vi "navX Example v2.vi"() -> ()   [LabVIEW 2015]
uses:
  navX Library v2/TypeDefs/Flags/Z900_navX_Flags_HardwareRevTypeDef.ctl
  navX Library v2/TypeDefs/Flags/Z900_navX_Flags_OmnimountConfigTypeDef.ctl
  navX Library v2/TypeDefs/Z900_navX_SerialStreamTypeDef.ctl
  NI WPI/WPI_SerialPort_USB.ctl
  <vilib>/Rock Robotics/SystemInterfaces/i2clib/i2c_bus.ctl
  <vilib>/Rock Robotics/SystemInterfaces/spilib/spi_bus.ctl
  navX Library v2/TypeDefs/Flags/Z900_navX_Flags_OpStatusTypeDef.ctl
  navX Library v2/TypeDefs/Flags/Z900_navX_Flags_CalibrationStatusTypeDef.ctl
  navX Library v2/IO/Open/Z900_navX_Open_Serial.vi
  navX Library v2/IO/Open/Z900_navX_Open_I2C.vi
  navX Library v2/IO/Open/Z900_navX_Open_SPI.vi
  navX Library v2/navX Library v2.lvlib
  NI WPI/NI WPI Serial USB.lvlib
panel:
  in  "Zero Displacement":bool
  out "Status":T3 {"OP Status" items=["INITIALIZING", "SELFTEST_IN_PROGRESS", "ERROR", "IMU_AUTOCAL_IN_PROGRESS", "NORMAL"]; "Calibration Status" items=["IMU_CAL_STATE_MASK"=3, "IMU_CAL_STATE_INPROGRESS"=0, "IMU_CAL_STATE_ACCUMULATE"=1, "IMU_CAL_STATE_COMPLETE"=2]}
  out "Connected":bool
  out "ERROR!":bool
  in  "Enable Logs":bool
  in  "Clear Log":bool
  out "Internal Error Log":errorcluster[](array[cluster])
  out "Log Size":i32
  in  "Interface Control":enum32{"Serial", "I2C", "SPI"}(tab)
  in  "Serial Port":T4=enum."MXP TTL"
  in  "Update Stream Type":bool
  in  "Stream Type":T5=enum."AHRS"
  in  "I2C Bus":T6=enum."I2C MXP"
  in  "SPI Bus":T7=enum."SPI MXP"
  in  "Clock Rate (Hz)":dbl=2000000.0 format="%_6f"
  in  "Zero Yaw":bool
  out "Raw Values":T8
  out "Quaternion":T9
  out "Linear Acceleration":T10
  out "Displacement":T11
  out "Offsets":T12
  out "Timestamp":u32
  out "MPUTemp":dbl(slide) scale=20.0..50.0
  in  "Update Rate":u8=50 min=4 max=60
  out "Board Information":T15 {"Board"."Hardware Revision" items=["navX-MXP"=33, "navX-Micro"=40]; "Omnimount Config" items=["DEFAULT", "X_UP", "X_DOWN", "Y_UP", "Y_DOWN", "Z_UP", "Z_DOWN"]}
  out "YRPHfH":T16
  in  "stop":bool
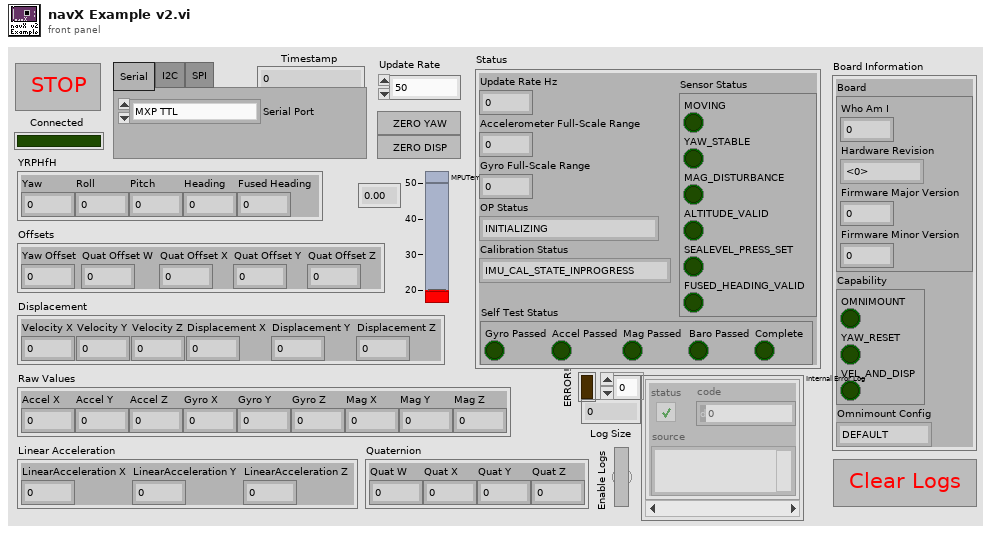
[diagram p1: front panel]
types:
  T1 = typedef "navX Library v2.lvlib/Z900_navX_Flags_OpStatusTypeDef.ctl" = u8
  T2 = typedef "navX Library v2.lvlib/Z900_navX_Flags_CalibrationStatusTypeDef.ctl" = u8
  T3 = cluster{"Update Rate Hz":u8, "Accelerometer Full-Scale Range":u8, "Gyro Full-Scale Range":u16, "OP Status":T1, "Calibration Status":T2, "Sensor Status":cluster{"MOVING":bool, "YAW_STABLE":bool, "MAG_DISTURBANCE":bool, "ALTITUDE_VALID":bool, "SEALEVEL_PRESS_SET":bool, "FUSED_HEADING_VALID":bool}, "Self Test Status":cluster{"Gyro Passed":bool, "Accel Passed":bool, "Mag Passed":bool, "Baro Passed":bool, "Complete":bool}}
  T4 = typedef "NI WPI Serial USB.lvlib/WPI_SerialPort_USB.ctl" = enum16{"Onboard RS-232", "MXP TTL", "USB"}
  T5 = typedef "navX Library v2.lvlib/Z900_navX_SerialStreamTypeDef.ctl" = enum16{"YRPH", "Quaterinons", "Gyro/Raw", "AHRS", "AHRSAndPositioning"}
  T6 = typedef "i2c_bus.ctl" = enum16{"I2C On-Board", "I2C MXP", "Invalid"}
  T7 = typedef "spi_bus.ctl" = enum16{"SPI On-Board, CS0", "SPI On-Board, CS1", "SPI On-Board, CS2", "SPI On-Board, CS3", "SPI MXP", "Invalid"}
  T8 = cluster{"Accel X":dbl, "Accel Y":dbl, "Accel Z":dbl, "Gyro X":dbl, "Gyro Y":dbl, "Gyro Z":dbl, "Mag X":dbl, "Mag Y":dbl, "Mag Z":dbl}
  T9 = cluster{"Quat W":dbl, "Quat X":dbl, "Quat Y":dbl, "Quat Z":dbl}
  T10 = cluster{"LinearAcceleration X":dbl, "LinearAcceleration Y":dbl, "LinearAcceleration Z":dbl}
  T11 = cluster{"Velocity X":dbl, "Velocity Y":dbl, "Velocity Z":dbl, "Displacement X":dbl, "Displacement Y":dbl, "Displacement Z":dbl}
  T12 = cluster{"Yaw Offset":dbl, "Quat Offset W":dbl, "Quat Offset X":dbl, "Quat Offset Y":dbl, "Quat Offset Z":dbl}
  T13 = typedef "navX Library v2.lvlib/Z900_navX_Flags_HardwareRevTypeDef.ctl" = u8
  T14 = typedef "navX Library v2.lvlib/Z900_navX_Flags_OmnimountConfigTypeDef.ctl" = u8
  T15 = cluster{"Board":cluster{"Who Am I":u8, "Hardware Revision":T13, "Firmware Major Version":u8, "Firmware Minor Version":u8}, "Capability":cluster{"OMNIMOUNT":bool, "YAW_RESET":bool, "VEL_AND_DISP":bool}, "Omnimount Config":T14}
  T16 = cluster{"Yaw":dbl, "Roll":dbl, "Pitch":dbl, "Heading":dbl, "Fused Heading":dbl}
  T17 = cluster{"Interface Control":enum32{"Serial", "I2C", "SPI"}, "Serial Port":T4, "I2C Bus":T6, "SPI Bus":T7, u8, "Clock Rate (Hz)":dbl}
  T18 = cluster{"Interface Control":bool, "Serial Port":bool, "I2C Bus":bool, "SPI Bus":bool, bool, "Clock Rate (Hz)":bool}
  T19 = typedef "navX Library v2.lvlib/Z900_navX_DeviceTypeDef.ctl" = cluster{"Interface":cluster{"Protocol":T20, "Update Rate (4Hz-100Hz)":u8, "navX Open TypeDef":variant}, "Notify Packet":refnum<notifier>, "Loop VI Refnum":refnum<vi>, "Ready to Close Occurrence Refnum":refnum<k4>}
  T20 = typedef "navX Library v2.lvlib/Z900_navX_ProtocolTypeDef.ctl" = enum16{"SERIAL", "I2C", "SPI"}
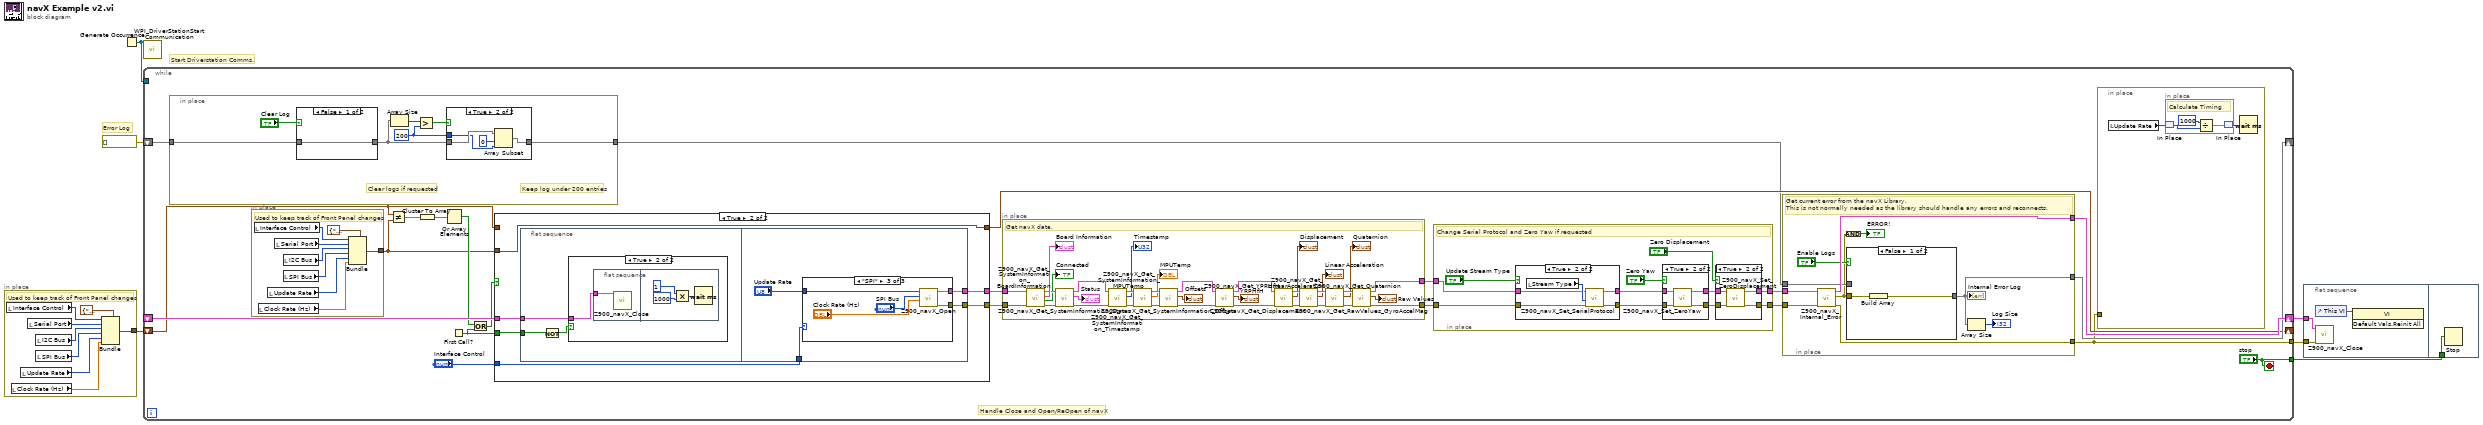
[diagram p0: block diagram]
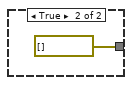
[diagram p3: hidden frame]
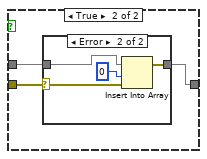
[diagram p4: hidden frame]
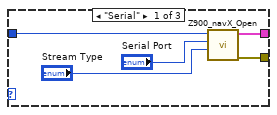
[diagram p11: hidden frame]
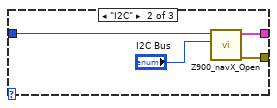
[diagram p12: hidden frame]
diagram:
  # "Start Driverstation Comms."
  # "Error Log"
  n1 = in-place {
    in-place-border: [w13] -> w3
    # "Used to keep track of Front Panel changes"
    n2 = local read "Interface Control"() -> (w12:enum32{"Serial", "I2C", "SPI"})
    n3 = local read "Clock Rate (Hz)"() -> (w7:dbl)
    n4 = local read "Update Rate"() -> (w8:u8)
    n5 = local read "Serial Port"() -> (w11:T4)
    n6 = local read "I2C Bus"() -> (w10:T6)
    n7 = local read "SPI Bus"() -> (w9:T7)
    n8 = Bundle(cluster=T17 {"Interface Control"=enum."Serial", "Serial Port"=enum."Onboard RS-232", "I2C Bus"=enum."I2C On-Board", "SPI Bus"=enum."SPI On-Board, CS0", 0, "Clock Rate (Hz)"=0.0} ("output cluster"), "Interface Control"=w12, "Serial Port"=w11, "I2C Bus"=w10, "SPI Bus"=w9, w8, "Clock Rate (Hz)"=w7) -> (w13:T17)
  }
  n9 = Generate Occurrence() -> (w2:refnum<k4>)
  n10 = call <vilib>:"WPI_DriverStationStart Communication.vi"("occurrence"=w2) -> ()  [unwired: 11 in]
  n11 = while {
    shift-right: [w32] -> w6
    shift-left: _ -> [w30]
    shift-right: [w31] -> _
    shift-left: errorcluster[] [] -> [w18]
    tunnel: [w15] -> w4
    shift-right: [w21] -> _
    shift-left: w3 -> [w20]
    tunnel: w2 -> [_]
    tunnel: ["stop"] -> w1
    stop <- "stop" stop-if-true
    # "Handle Close and Open/ReOpen of navX"
    n12 = in-place {
      in-place-border: w18 -> [w56]
      in-place-border: [w52] -> w17
      w51 = 200 ("y")
      # "Clear logs if requested"
      # "Keep log under 200 entries"
      n13 = case shown="False" "Clear Log" {
        tunnel: [w62 errorcluster[] []] -> w50
        tunnel: w56 -> [w62 _]
        frame False {
        }
        frame True {
        }
      }
      n14 = Array Size(array=w50) -> (size(s)=w55:i32)
      n15 = Greater?(x=w55, y=w51) -> (0:w53:bool)
      n16 = case shown="True" w53 {
        tunnel: [w57 w58] -> w52
        tunnel: w50 -> [w57 w61]
        tunnel: w51 -> [_ w59]
        frame False {
        }
        frame True {
          n17 = Array Subset(array=w61, index=0, length=w59) -> (w58:errorcluster[])
        }
      }
    }
    n18 = in-place {
      in-place-border: [w48] -> w16
      # "Used to keep track of Front Panel changes"
      n19 = local read "Interface Control"() -> (w47:enum32{"Serial", "I2C", "SPI"})
      n20 = local read "Clock Rate (Hz)"() -> (w42:dbl)
      n21 = local read "Update Rate"() -> (w43:u8)
      n22 = local read "Serial Port"() -> (w46:T4)
      n23 = local read "I2C Bus"() -> (w45:T6)
      n24 = local read "SPI Bus"() -> (w44:T7)
      n25 = Bundle(cluster=T17 {"Interface Control"=enum."Serial", "Serial Port"=enum."Onboard RS-232", "I2C Bus"=enum."I2C On-Board", "SPI Bus"=enum."SPI On-Board, CS0", 0, "Clock Rate (Hz)"=0.0} ("output cluster"), "Interface Control"=w47, "Serial Port"=w46, "I2C Bus"=w45, "SPI Bus"=w44, w43, "Clock Rate (Hz)"=w42) -> (w48:T17)
    }
    n26 = Not Equal?(x=w20, y=w16) -> (x != y?=w24:T18)
    n27 = Cluster To Array(cluster=w24) -> (array=w23:bool[])
    n28 = Or Array Elements(Boolean array=w23) -> (logical OR=w22:bool)
    n29 = First Call?() -> (First Call?: T/F=w26:bool)
    n30 = Or(x=w22, y=w26) -> (x .or. y?=w27:bool)
    n31 = case shown="True" w27 {
      tunnel: w30 -> [w148 w154]
      tunnel: [w148 w149] -> w29
      tunnel: [_ w153] -> w28
      tunnel: "Interface Control" -> [_ w152]
      tunnel: w26 -> [_ w151]
      tunnel: w16 -> [_ w150]
      tunnel: [w147 w150] -> w21
      tunnel: w20 -> [w147 _]
      frame False {
      }
      frame True {
        n32 = flat-sequence {
          tunnel: w151 -> [w155]
          tunnel: w154 -> [w156]
          tunnel: [w165] -> w149
          tunnel: [w164] -> w153
          tunnel: w152 -> [w163]
          frame #0 {
            n33 = Not(x=w155) -> (.not. x?=w157:bool)
            n34 = case shown="True" w157 {
              tunnel: w156 -> [_ w158]
              frame False {
              }
              frame True {
                n35 = flat-sequence {
                  tunnel: w158 -> [w159]
                  frame #0 {
                    n36 = call "Z900_navX_Close.vi"("navX Device"=w159) -> ()  [unwired: 10 in, 1 out]
                  }
                  frame #1 {
                    n37 = Multiply(x=u32 1, y=u32 1000 ("x")) -> (x*y=w161:u32)
                    n38 = Wait (ms)(milliseconds to wait=w161) -> ()  [unwired: 1 out]
                  }
                }
              }
            }
          }
          frame #1 {
            n39 = case shown="\"SPI\"" w163 {
              tunnel: [w169 w173 w179] -> w165
              tunnel: [w168 w172 w178] -> w164
              tunnel: "Update Rate" -> [w167 w175 w177]
              frame "Serial" {
                n40 = call-poly "Z900_navX_Open.vi"("Stream Type"="Stream Type", "Serial Port"="Serial Port", "Update Rate (4Hz-60Hz)"=w167) -> ("error out"=w168:errorcluster, "navX Device"=w169:T19)  [unwired: 7 in]
              }
              frame "I2C" {
                n41 = call-poly "Z900_navX_Open.vi"("I2C Bus"="I2C Bus", "Update Rate (4Hz-60Hz)"=w175) -> ("error out"=w172:errorcluster, "navX Device"=w173:T19)  [unwired: 8 in]
              }
              frame "SPI" {
                n42 = call-poly "Z900_navX_Open.vi"("Clock Rate (Hz)"="Clock Rate (Hz)", "SPI Bus"="SPI Bus", "Update Rate (4Hz-60Hz)"=w177) -> ("error out"=w178:errorcluster, "navX Device"=w179:T19)  [unwired: 7 in]
              }
            }
          }
        }
      }
    }
    n43 = in-place {
      in-place-border: [w119] -> w36
      in-place-border: [w118] -> w35
      in-place-border: w29 -> [w117]
      in-place-border: w28 -> [w116]
      # "Get navX data."
      n44 = call "Z900_navX_Get_SystemInformation_BoardInformation.vi"("error in (no error)"=w116, "navX Device"=w117) -> ("error out"=w144:errorcluster, "Connected"=→"Connected":bool, "Board Information"=→"Board Information":T15, "navX Device"=w143:T19)  [unwired: 6 in]
      n45 = call "Z900_navX_Get_SystemInformation_Status.vi"("error in (no error)"=w144, "navX Device"=w143) -> ("error out"=w142:errorcluster, "Status"=→"Status":T3, "navX Device"=w141:T19)  [unwired: 6 in, 1 out]
      n46 = call "Z900_navX_Get_SystemInformation_Timestamp.vi"("error in (no error)"=w142, "navX Device"=w141) -> ("error out"=w139:errorcluster, "Timestamp"=→"Timestamp":u32, "navX Device"=w140:T19)  [unwired: 6 in, 1 out]
      n47 = call "Z900_navX_Get_SystemInformation_MPUTemp.vi"("error in (no error)"=w139, "navX Device"=w140) -> ("error out"=w137:errorcluster, "MPUTemp"=→"MPUTemp":dbl, "navX Device"=w138:T19)  [unwired: 6 in, 1 out]
      n48 = call "Z900_navX_Get_SystemInformation_Offsets.vi"("error in (no error)"=w137, "navX Device"=w138) -> ("error out"=w135:errorcluster, "Offsets"=→"Offsets":T12, "navX Device"=w136:T19)  [unwired: 6 in, 1 out]
      n49 = call "Z900_navX_Get_YPRHfH.vi"("error in (no error)"=w135, "navX Device"=w136) -> ("error out"=w133:errorcluster, "YRPHfH"=→"YRPHfH":T16, "navX Device"=w134:T19)  [unwired: 6 in, 1 out]
      n50 = call "Z900_navX_Get_Displacement.vi"("error in (no error)"=w133, "navX Device"=w134) -> ("error out"=w131:errorcluster, "Displacement"=→"Displacement":T11, "navX Device"=w132:T19)  [unwired: 6 in, 1 out]
      n51 = call "Z900_navX_Get_LinearAcceleration.vi"("error in (no error)"=w131, "navX Device"=w132) -> ("error out"=w129:errorcluster, "Linear Acceleration"=→"Linear Acceleration":T10, "navX Device"=w130:T19)  [unwired: 6 in, 1 out]
      n52 = call "Z900_navX_Get_Quaternion.vi"("error in (no error)"=w129, "navX Device"=w130) -> ("error out"=w127:errorcluster, "Quaternion"=→"Quaternion":T9, "navX Device"=w128:T19)  [unwired: 6 in, 1 out]
      n53 = call "Z900_navX_Get_RawValues_GyroAccelMag.vi"("error in (no error)"=w127, "navX Device"=w128) -> ("error out"=w118:errorcluster, "Raw Values"=→"Raw Values":T8, "navX Device"=w119:T19)  [unwired: 6 in, 1 out]
    }
    n54 = in-place {
      in-place-border: w36 -> [w94]
      in-place-border: w35 -> [w93]
      in-place-border: [w86] -> w34
      in-place-border: [w85] -> w33
      # "Change Serial Protocol and Zero Yaw if requested"
      n55 = case shown="True" "Update Stream Type" {
        tunnel: w94 -> [w108 w112]
        tunnel: [w108 w111] -> w92
        tunnel: w93 -> [w107 w110]
        tunnel: [w107 w109] -> w91
        frame False {
        }
        frame True {
          n56 = local read "Stream Type"() -> (w113:T5)
          n57 = call "Z900_navX_Set_SerialProtocol.vi"("error in (no error)"=w110, "Stream Type"=w113, "navX Device"=w112) -> ("error out"=w109:errorcluster, "navX Device"=w111:T19)  [unwired: 7 in]
        }
      }
      n58 = case shown="True" "Zero Yaw" {
        tunnel: w92 -> [w102 w106]
        tunnel: [w102 w105] -> w88
        tunnel: w91 -> [w101 w104]
        tunnel: [w101 w103] -> w87
        frame False {
        }
        frame True {
          n59 = call "Z900_navX_Set_ZeroYaw.vi"("error in (no error)"=w104, "navX Device"=w106) -> ("error out"=w103:errorcluster, "navX Device"=w105:T19)  [unwired: 8 in]
        }
      }
      n60 = case shown="True" "Zero Displacement" {
        tunnel: w88 -> [w96 w100]
        tunnel: [w96 w99] -> w86
        tunnel: w87 -> [w95 w98]
        tunnel: [w95 w97] -> w85
        frame False {
        }
        frame True {
          n61 = call "Z900_navX_Set_ZeroDisplacement.vi"("error in (no error)"=w98, "navX Device"=w100) -> ("error out"=w97:errorcluster, "navX Device"=w99:T19)  [unwired: 8 in]
        }
      }
    }
    n62 = in-place {
      in-place-border: w34 -> [w73]
      in-place-border: w33 -> [w72]
      in-place-border: [w71] -> w32
      in-place-border: [w70] -> w31
      in-place-border: [w68] -> w15
      in-place-border: w17 -> [w66]
      # "Get current error from the navX Library.\nThis is not normally needed as the library should handle any errors and reconnects."
      n63 = call "Z900_navX_Internal_Error.vi"("error in (no error)"=w72, "navX Device"=w73) -> ("error out"=w68:errorcluster, "Internal error out"=w65:errorcluster, "navX Device"=w71:T19)  [unwired: 7 in]
      n64 = Compound Arithmetic op=AND(w65) -> (→"ERROR!":bool)
      n65 = case shown="False" "Enable Logs" {
        tunnel: w65 -> [w75 w78]
        tunnel: [w74 w77] -> w70
        tunnel: w66 -> [_ w76]
        frame False {
          n66 = Build Array(w75) -> (w74:errorcluster[])
        }
        frame True {
          n67 = case shown="Error" w78 {
            selector: w78 -> [_ w82]
            tunnel: [w79 w80] -> w77
            tunnel: w76 -> [w79 w83]
            frame No Error {
            }
            frame Error {
              n68 = Insert Into Array(array=w83, index=0, new element=w82) -> (w80:errorcluster[])
            }
          }
        }
      }
      "Internal Error Log" <- w70
      n69 = Array Size(array=w70) -> (size(s)=→"Log Size":i32)
    }
    n70 = in-place {
      in-place-border: w15 -> [_]
      n71 = local read "Update Rate"() -> (w38:u8)
      n72 = in-place {
        # "Calculate Timing"
        n73 = in-place-match #1(w38) -> (w40:u8)
        n74 = Divide(x=1000, y=w40) -> (x/y=w39:dbl)
        n75 = in-place-match #1(w39) -> (w37:u8)
      }
      n76 = Wait (ms)(milliseconds to wait=w37) -> ()  [unwired: 1 out]
    }
  }
  n77 = flat-sequence {
    tunnel: w6 -> [w183]
    tunnel: w4 -> [w182]
    tunnel: w1 -> [w184]
    frame #0 {
      n78 = control-ref of="This VI"() -> (w181:refnum<vi>)
      n79 = call "Z900_navX_Close.vi"("error in (no error)"=w182, "navX Device"=w183) -> ()  [unwired: 9 in, 1 out]
      n80 = invoke class="VI" method="Default Vals.Reinit All"(reference=w181) -> ()  [unwired: 2 in, 3 out]
    }
    frame #1 {
      n81 = Stop(stop? (T)=w184) -> ()
    }
  }
